vi "Globale Variable.vi"() -> ()   [LabVIEW 2016]
panel:
  out "Ta0":dbl
  out "b":dbl
  out "a":dbl
  out "r_lqr":dbl
  out "q_lqr":dbl
  out "launch button":bool
  out "v_erod > v_max":bool
  out "ready to log!":bool
  out "manual Gain":bool
  out "voltage_start":dbl
  out "starting threshhold":dbl
  out "v_max":dbl
  out "lambda_target":dbl
  out "enable controlled throttle --> blue light":bool
  out "lambda error":dbl
  out "vHL":dbl
  out "vHR":dbl
  out "throttle voltage":dbl
  out "k_lqr":dbl
  out "lambda":dbl
  out "vVL":dbl
  out "v_rear":dbl
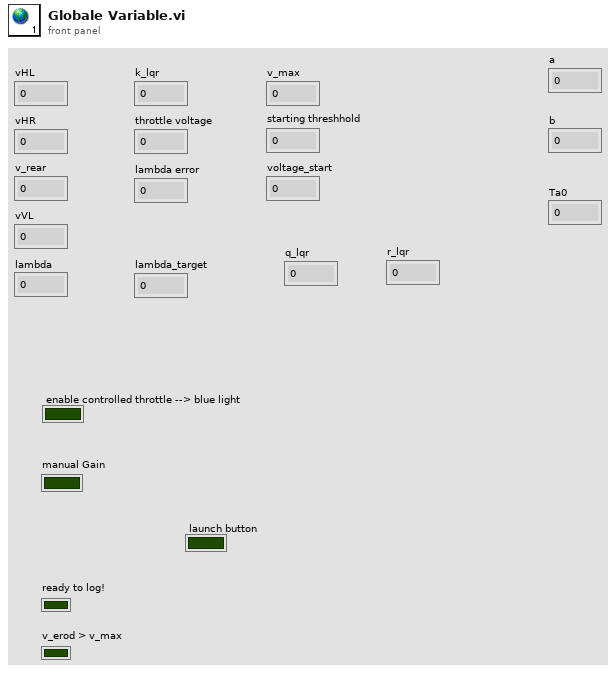
[diagram p1: front panel]
diagram:
